vi "UpdatePulseType.vi"(1 "Sham stimulations:":i32=1 min=0, 2 "Real stimulations:":i32=1 min=1) -> (0 "Real stim on":bool)   [LabVIEW 2017]
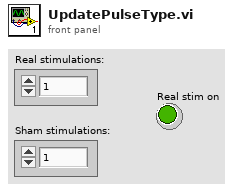
[diagram p1: front panel]
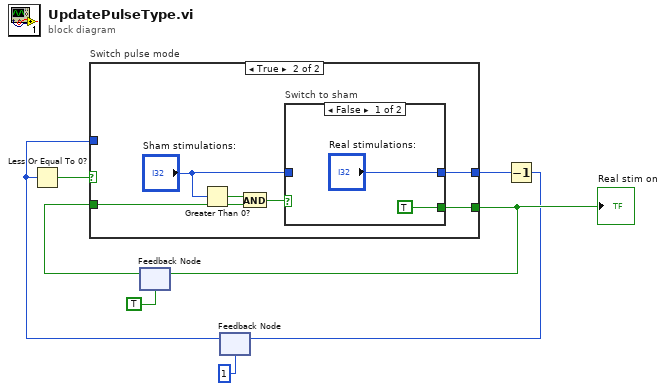
[diagram p0: block diagram]
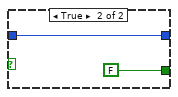
[diagram p3: hidden frame]
diagram:
  n1 = feedback #1 ("Real stim on")(TRUE) -> (w6:bool)
  n2 = feedback #2(1) -> (w3:i32)
  n3 = Less Or Equal To 0?(x=w3) -> (x <= 0?=w8:bool)
  n4 = case "Switch pulse mode" shown="True" w8 {
    tunnel: w3 -> [w10 _]
    tunnel: [w10 w13] -> w2
    tunnel: [w9 w12] -> w5
    tunnel: w6 -> [w9 w11]
    frame False {
    }
    frame True {
      n5 = Greater Than 0?(x="Sham stimulations:") -> (x > 0?=w16:bool)
      n6 = And(x=w16, y=w11) -> (x .and. y?=w15:bool)
      n7 = case "Switch to sham" shown="False" w15 {
        tunnel: "Sham stimulations:" -> [_ w20]
        tunnel: ["Real stimulations:" w20] -> w13
        tunnel: [TRUE FALSE] -> w12
        frame False {
        }
        frame True {
        }
      }
    }
  }
  "Real stim on" <- w5
  n8 = feedback-in #1(w5) -> ()
  n9 = Decrement(x=w2) -> (x-1=w1:i32)
  n10 = feedback-in #2(w1) -> ()
